vi "pressure_units.vi"() -> ()   [LabVIEW 2010]
panel:
  out "Converted Value":dbl
  in  "Input Value:":dbl
  in  "Output Pressure Units":T1(radio)
  in  "Input Pressure Units":T1(radio)
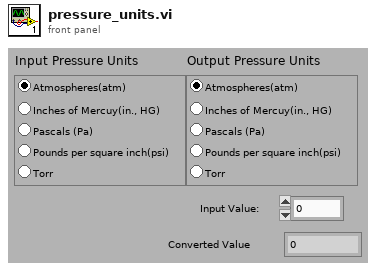
[diagram p1: front panel]
types:
  T1 = enum32{"Atmospheres(atm)", "Inches of Mercuy(in., HG)", "Pascals (Pa)", "Pounds per square inch(psi)", "Torr"}
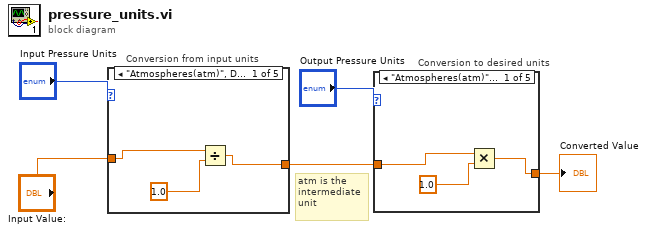
[diagram p0: block diagram]
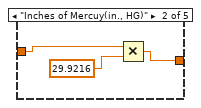
[diagram p2: hidden frame]
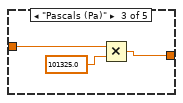
[diagram p3: hidden frame]
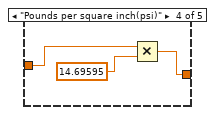
[diagram p4: hidden frame]
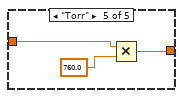
[diagram p5: hidden frame]
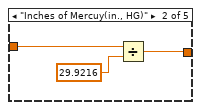
[diagram p6: hidden frame]
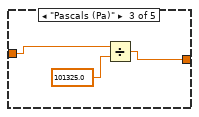
[diagram p7: hidden frame]
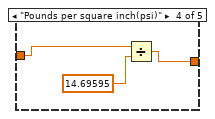
[diagram p8: hidden frame]
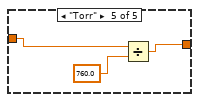
[diagram p9: hidden frame]
diagram:
  # "atm is the intermediate unit"
  n1 = case "Conversion from input units" shown="\"Atmospheres(atm)\", Default" "Input Pressure Units" {
    tunnel: "Input Value:" -> [w6 w10 w14 w16 w19]
    tunnel: [w7 w9 w12 w15 w18] -> w1
    frame "Atmospheres(atm)", Default {
      n2 = Divide(x=w6, y=1.0) -> (x/y=w7:dbl)
    }
    frame "Inches of Mercuy(in., HG)" {
      n3 = Divide(x=w10, y=29.9216) -> (x/y=w9:dbl)
    }
    frame "Pascals (Pa)" {
      n4 = Divide(x=w14, y=101325.0) -> (x/y=w12:dbl)
    }
    frame "Pounds per square inch(psi)" {
      n5 = Divide(x=w16, y=14.69595) -> (x/y=w15:dbl)
    }
    frame "Torr" {
      n6 = Divide(x=w19, y=760.0) -> (x/y=w18:dbl)
    }
  }
  n7 = case "Conversion to desired units" shown="\"Atmospheres(atm)\", Default" "Output Pressure Units" {
    tunnel: [w22 w24 w28 w31 w35] -> w3
    tunnel: w1 -> [w21 w26 w27 w30 w33]
    frame "Atmospheres(atm)", Default {
      n8 = Multiply(x=w21, y=1.0) -> (x*y=w22:dbl)
    }
    frame "Inches of Mercuy(in., HG)" {
      n9 = Multiply(x=w26, y=29.9216) -> (x*y=w24:dbl)
    }
    frame "Pascals (Pa)" {
      n10 = Multiply(x=w27, y=101325.0) -> (x*y=w28:dbl)
    }
    frame "Pounds per square inch(psi)" {
      n11 = Multiply(x=w30, y=14.69595) -> (x*y=w31:dbl)
    }
    frame "Torr" {
      n12 = Multiply(x=w33, y=760.0) -> (x*y=w35:dbl)
    }
  }
  "Converted Value" <- w3
